vi "Select Screen Page.vi"(8 "error in (no error)":errorcluster, 10 "Screen Page":u16(ring) items=["Setup", "Channel", "Trigger", "Scope", "Replay"], 11 "VISA resource name":refnum<visa-resource-name>) -> (0 "error out":errorcluster, 3 "VISA resource name out":refnum<visa-resource-name>)   [LabVIEW 2017, in "Sefram DAS220.lvlib"]
doc: "Change the current page displayed on the device."
uses:
  <instrlib>/Sefram DAS220/Sefram DAS220.lvlib
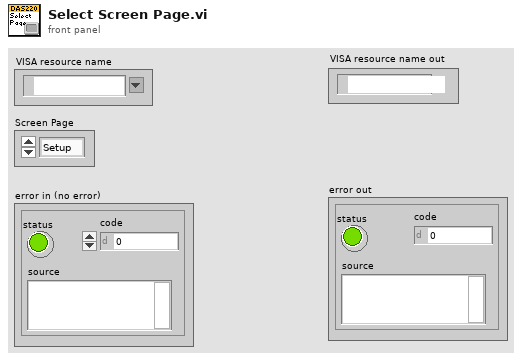
[diagram p1: front panel]
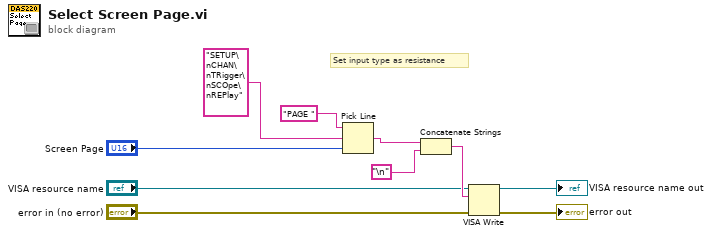
[diagram p0: block diagram]
diagram:
  # "Set input type as resistance"
  n1 = Pick Line(string ("")="PAGE " ("string"), multi-line string="SETUP\nCHAN\nTRigger\nSCOpe\nREPlay", line index="Screen Page") -> (output string=w4:string)
  n2 = Concatenate Strings(w4, "\n") -> (w10:string)
  n3 = VISA Write(VISA resource name="VISA resource name", write buffer=w10, error in (no error)="error in (no error)") -> (VISA resource name out=→"VISA resource name out":refnum<visa-resource-name>, error out=→"error out":errorcluster)  [unwired: 1 out]
